vi "DoubleCoincidencesCheck_write_delay.vi"(11 "Cluster In in":T1 {"Coincidence Window" format="%#_13g"; "Delay12" format="%#_13g"; "Delay02" format="%#_13g"; "Delay01" format="%#_13g"}) -> (3 "Cluster In out":T1 {"Coincidence Window" format="%#_13g"; "Delay12" format="%#_13g"; "Delay02" format="%#_13g"; "Delay01" format="%#_13g"})   [LabVIEW 2023]
uses:
  Get_Delays_Ctrl.ctl
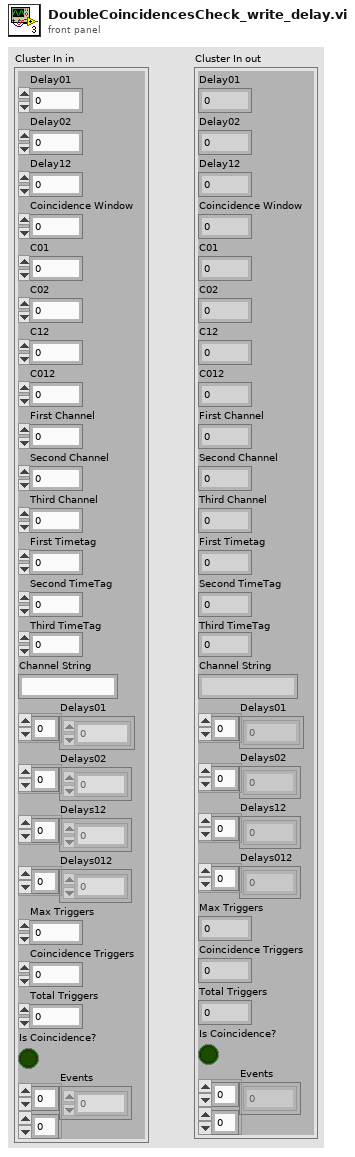
[diagram p1: front panel]
types:
  T1 = typedef "Get_Delays_Ctrl.ctl" = cluster{"Delay01":dbl, "Delay02":dbl, "Delay12":dbl, "Coincidence Window":dbl, "C01":u32, "C02":u32, "C12":u32, "C012":u32, "First Channel":dbl, "Second Channel":dbl, "Third Channel":dbl, "First Timetag":dbl, "Second TimeTag":dbl, "Third TimeTag":dbl, "Channel String":string, "Delays01":sgl[], "Delays02":dbl[], "Delays12":dbl[], "Delays012":dbl[], "Max Triggers":i32, "Coincidence Triggers":i32, "Total Triggers":i32, "Is Coincidence?":bool, "Events":u64[][]}
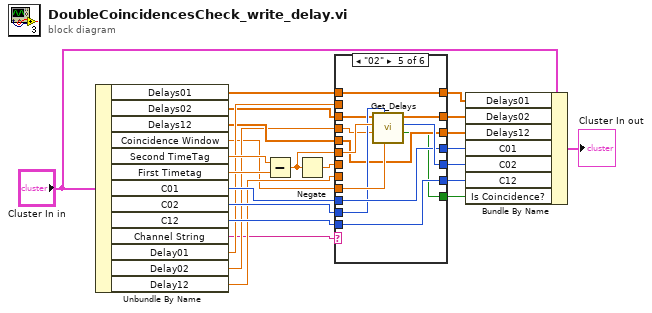
[diagram p0: block diagram]
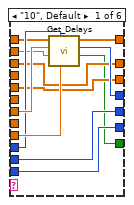
[diagram p2: hidden frame]
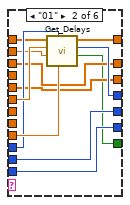
[diagram p3: hidden frame]
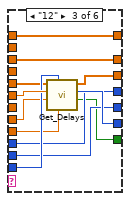
[diagram p4: hidden frame]
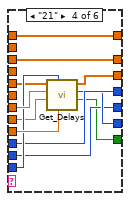
[diagram p5: hidden frame]
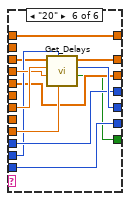
[diagram p6: hidden frame]
diagram:
  n1 = Unbundle By Name("Cluster In in") -> ("Delays01"=w13:sgl[], "Delays02"=w14:dbl[], "Delays12"=w17:dbl[], "Coincidence Window"=w12:dbl, "Second TimeTag"=w20:dbl, "First Timetag"=w21:dbl, "C01"=w23:u32, "C02"=w24:u32, "C12"=w22:u32, "Channel String"=w15:string, "Delay01"=w19:dbl, "Delay02"=w16:dbl, "Delay12"=w18:dbl)
  n2 = Subtract(x=w20, y=w21) -> (x-y=w10:dbl)
  n3 = Negate(x=w10) -> (-x=w11:dbl)
  n4 = case shown="\"02\"" w15 {
    tunnel: w10 -> [_ w48 w60 _ w84 _]
    tunnel: w11 -> [w36 _ _ w72 _ w95]
    tunnel: [w34 w47 w51 w63 w75 w90] -> w3
    tunnel: [w27 w39 w50 w62 w83 w96] -> w2
    tunnel: [w26 w38 w59 w70 w74 w87] -> w1
    tunnel: w13 -> [w29 w41 w51 w63 w75 w90]
    tunnel: w14 -> [w27 w39 w50 w62 w77 w86]
    tunnel: w12 -> [w35 w46 w57 w71 w81 w94]
    tunnel: [w31 w43 w55 w66 w82 w93] -> w6
    tunnel: w23 -> [w33 w45 w54 w68 w79 w92]
    tunnel: w22 -> [w30 w42 w58 w69 w80 w91]
    tunnel: [w32 w44 w54 w68 w79 w92] -> w4
    tunnel: w24 -> [w31 w43 w55 w66 w78 w88]
    tunnel: [w30 w42 w56 w67 w80 w91] -> w5
    tunnel: w16 -> [_ _ _ _ w76 w89]
    tunnel: w17 -> [w26 w38 w53 w65 w74 w87]
    tunnel: w18 -> [_ _ w52 w64 _ _]
    tunnel: w19 -> [w28 w40 _ _ _ _]
    tunnel: [w25 w37 w49 w61 w73 w85] -> w9
    frame "10", Default {
      n5 = call "Get_Delays.vi"("Coincidence Window"=w35, "Coincidences In"=w33, "Expected Delay"=w28, "Delay"=w36, "Delays In"=w29) -> ("Is Coincidence?"=w25:bool, "Coincidences out"=w32:u32, "Delays Out"=w34:dbl[])  [unwired: 4 in]
    }
    frame "01" {
      n6 = call "Get_Delays.vi"("Coincidence Window"=w46, "Coincidences In"=w45, "Expected Delay"=w40, "Delay"=w48, "Delays In"=w41) -> ("Is Coincidence?"=w37:bool, "Coincidences out"=w44:u32, "Delays Out"=w47:dbl[])  [unwired: 4 in]
    }
    frame "12" {
      n7 = call "Get_Delays.vi"("Coincidence Window"=w57, "Coincidences In"=w58, "Expected Delay"=w52, "Delay"=w60, "Delays In"=w53) -> ("Is Coincidence?"=w49:bool, "Coincidences out"=w56:u32, "Delays Out"=w59:dbl[])  [unwired: 4 in]
    }
    frame "21" {
      n8 = call "Get_Delays.vi"("Coincidence Window"=w71, "Coincidences In"=w69, "Expected Delay"=w64, "Delay"=w72, "Delays In"=w65) -> ("Is Coincidence?"=w61:bool, "Coincidences out"=w67:u32, "Delays Out"=w70:dbl[])  [unwired: 4 in]
    }
    frame "02" {
      n9 = call "Get_Delays.vi"("Coincidence Window"=w81, "Coincidences In"=w78, "Expected Delay"=w76, "Delay"=w84, "Delays In"=w77) -> ("Is Coincidence?"=w73:bool, "Coincidences out"=w82:u32, "Delays Out"=w83:dbl[])  [unwired: 4 in]
    }
    frame "20" {
      n10 = call "Get_Delays.vi"("Coincidence Window"=w94, "Coincidences In"=w88, "Expected Delay"=w89, "Delay"=w95, "Delays In"=w86) -> ("Is Coincidence?"=w85:bool, "Coincidences out"=w93:u32, "Delays Out"=w96:dbl[])  [unwired: 4 in]
    }
  }
  n11 = Bundle By Name(cluster="Cluster In in", "Delays01"=w3, "Delays02"=w2, "Delays12"=w1, "C01"=w4, "C02"=w6, "C12"=w5, "Is Coincidence?"=w9) -> (→"Cluster In out":T1)
